vi "Image_Crop.vi"(6 "Crop?":bool, 8 "error in":errorcluster, 10 "Image In":T3, 11 "Camera":T1) -> (0 "error out":errorcluster, 2 "Image Out":T3)   [LabVIEW 2019]
uses:
  <vilib>/vision/Image Controls.llb/IMAQ Image.ctl
  Camera_ID.ctl
panel:
  in  "ROI Descriptor (Cam2)":T2={"Global Rectangle"=[715, 80, 1135, 1150], "Contours"=[{"ID"=enum."External", "Type"=3, "Coordinates"=[715, 0, 1135, 1150]}]} {"Contours"."Type" items=["No Selection", "Point", "Line", "Rectangle", "Oval", "Polygon", "Freehand Region", "Annulus", "Unused2", "Unused3", "Broken Line", "Freehand Line", "Rotated Rectangle"]}
  in  "ROI Descriptor (Cam1)":T2={"Global Rectangle"=[680, 170, 1100, 1150], "Contours"=[{"ID"=enum."External", "Type"=3, "Coordinates"=[680, 170, 1100, 1150]}]} {"Contours"."Type" items=["No Selection", "Point", "Line", "Rectangle", "Oval", "Polygon", "Freehand Region", "Annulus", "Unused2", "Unused3", "Broken Line", "Freehand Line", "Rotated Rectangle"]}
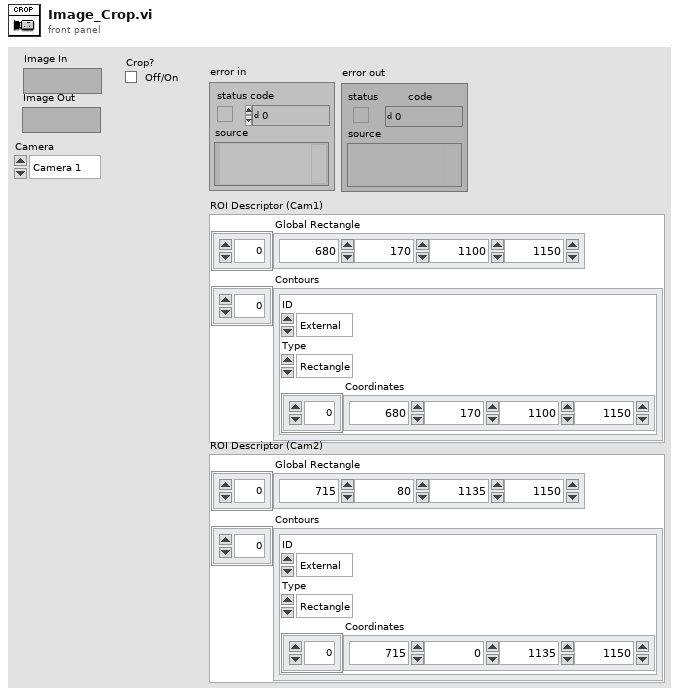
[diagram p1: front panel]
types:
  T1 = typedef "Camera_ID.ctl" = enum16{"Camera 1", "Camera 2"}
  T2 = cluster{"Global Rectangle":i32[], "Contours":cluster{"ID":enum32{"External", "Internal"}, "Type":u32, "Coordinates":i32[]}[]}
  T3 = typedef "IMAQ Image.ctl" = refnum<image>
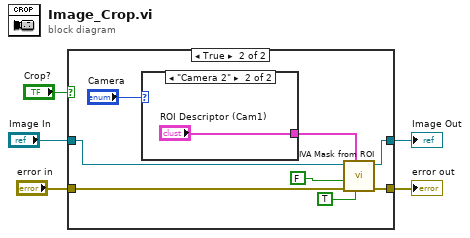
[diagram p0: block diagram]
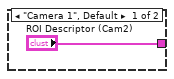
[diagram p3: hidden frame]
diagram:
  n1 = case shown="True" "Crop?" {
    tunnel: [w7 w15] -> w5
    tunnel: [w6 w14] -> w4
    tunnel: "Image In" -> [w7 w11]
    tunnel: "error in" -> [w6 w10]
    frame False {
    }
    frame True {
      n2 = case shown="\"Camera 2\"" "Camera" {
        tunnel: ["ROI Descriptor (Cam2)" "ROI Descriptor (Cam1)"] -> w8
        frame "Camera 1", Default {
        }
        frame "Camera 2" {
        }
      }
      n3 = call <vilib>:"IVA Mask from ROI.vi"("Shrink"=TRUE, "ROI Descriptor"=w8, "error in (no error)"=w10, "Out / In"=FALSE, "Image Src"=w11) -> ("error out"=w14:errorcluster, "Image Out"=w15:T3)  [unwired: 5 out]
    }
  }
  "error out" <- w4
  "Image Out" <- w5
